vi "EXECUTION_UI_INIT.vi"(5 "Show Panel Label":bool, 7 "Layout":T1, 8 "error in (no error)":errorcluster, 10 "Execution Panels":refnum<vi>[](array[refnum]), 11 "Container Panel":refnum<vi>) -> (0 "error out":errorcluster, 2 "Execution Panels In Use":refnum<vi>[](array[refnum]))   [LabVIEW 2015, in "Execution.lvclass"]
uses:
  Execution.lvclass
  <vilib>/Utility/miscctls.llb/LVPointTypeDef.ctl
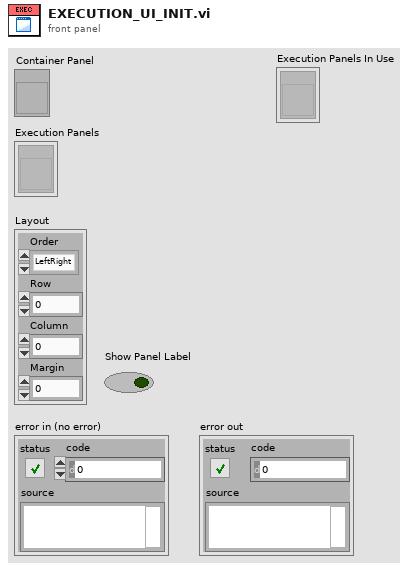
[diagram p1: front panel]
types:
  T1 = cluster{"Order":enum16{"LeftRight", "TopDown"}, "Row":i32, "Column":i32, "Margin":i32}
  T2 = enum16{"No Scaling", "Scale All Objects", "Scale Single Object"}
  T3 = typedef "LVPointTypeDef.ctl" = cluster{"Horizontal":i16, "Vertical":i16}
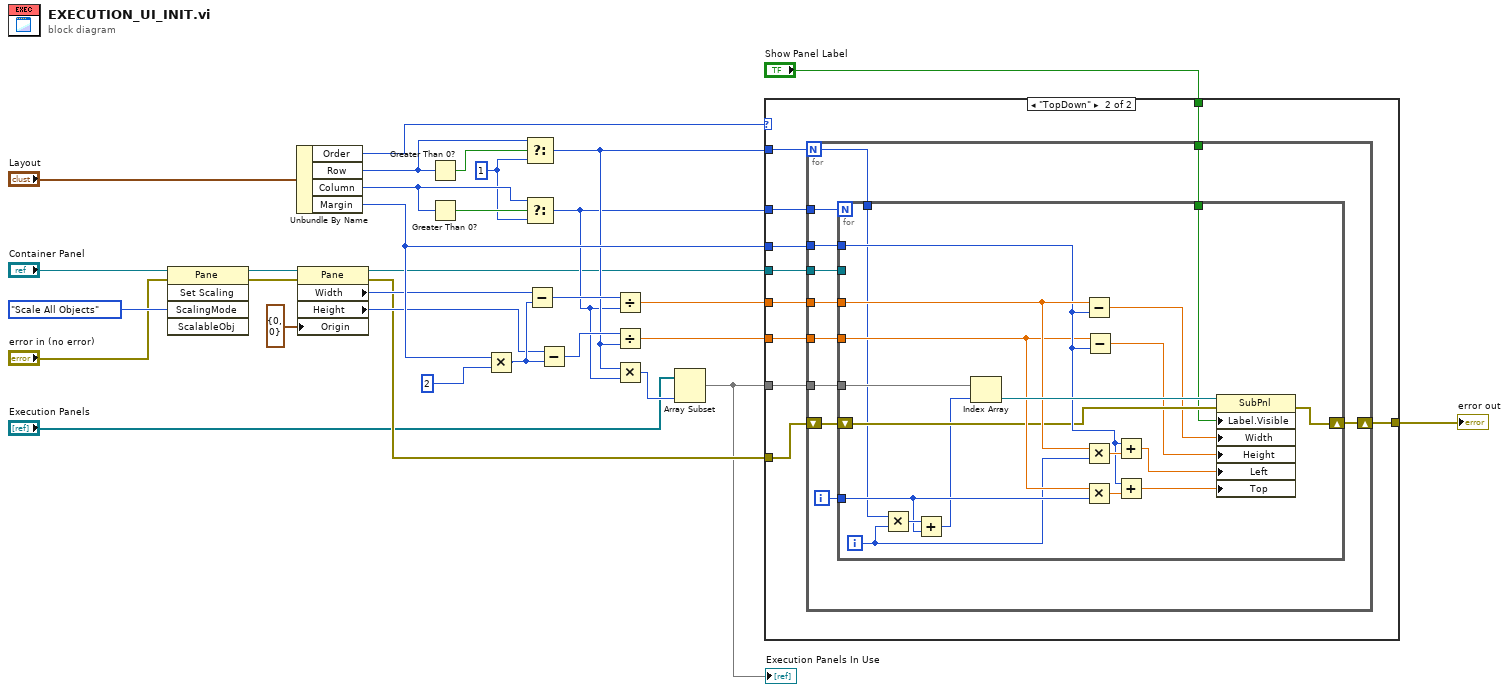
[diagram p0: block diagram]
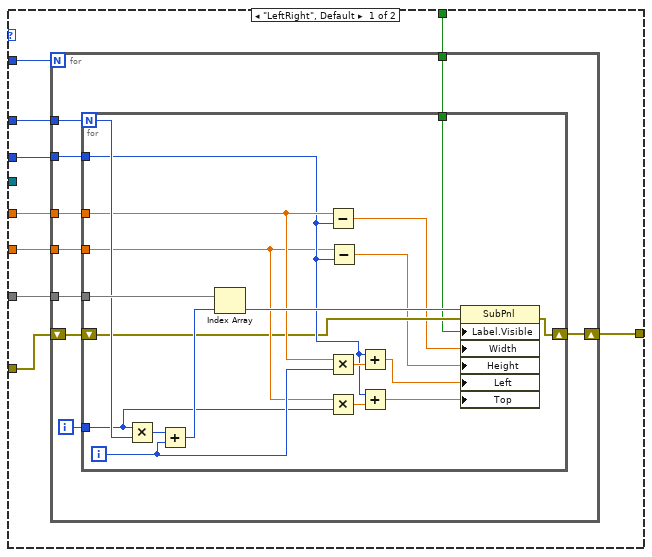
[diagram p2: hidden frame]
diagram:
  w13 = 1
  n1 = invoke class="Pane" method="Set Scaling"(reference="Container Panel", error in="error in (no error)", "ScalingMode"=T2."Scale All Objects" ("Scaling Mode")) -> (reference out=w2:refnum<vi>, error out=w3:errorcluster)  [unwired: 2 in, 3 out]
  n2 = Unbundle By Name("Layout") -> ("Order"=w30:enum16{"LeftRight", "TopDown"}, "Row"=w16:i32, "Column"=w14:i32, "Margin"=w31:i32)
  n3 = property class="Pane"(reference=w2, error in=w3, "Origin"=T3 {"Horizontal"=0, "Vertical"=0}) -> (reference out=w7:refnum<vi>, error out=w18:errorcluster, "Width"=w25:u32, "Height"=w26:u32)
  n4 = Greater Than 0?(x=w16) -> (x > 0?=w17:bool)
  n5 = Greater Than 0?(x=w14) -> (x > 0?=w15:bool)
  n6 = Multiply(x=w31, y=2) -> (x*y=w27:i32)
  n7 = Select(t=w16, s=w17, f=w13) -> (s? t:f=w12:i32)
  n8 = Select(t=w14, s=w15, f=w13) -> (s? t:f=w11:i32)
  n9 = Subtract(x=w25, y=w27) -> (x-y=w23:u32)
  n10 = Subtract(x=w26, y=w27) -> (x-y=w22:u32)
  n11 = Divide(x=w23, y=w11) -> (x/y=w19:dbl)
  n12 = Divide(x=w22, y=w12) -> (x/y=w20:dbl)
  n13 = Multiply(x=w12, y=w11) -> (x*y=w9:i32)
  n14 = Array Subset(array="Execution Panels", length=w9) -> (w10:refnum<vi>[])  [unwired: 1 in]
  "Execution Panels In Use" <- w10
  n15 = case shown="\"TopDown\"" w30 {
    tunnel: w19 -> [w40 w78]
    tunnel: w20 -> [w39 w77]
    tunnel: [w38 w76] -> w21
    tunnel: w10 -> [w37 w75]
    tunnel: w12 -> [w36 w74]
    tunnel: w11 -> [w35 w73]
    tunnel: w31 -> [w34 w72]
    tunnel: w18 -> [w33 w71]
    tunnel: "Show Panel Label" -> [w32 w70]
    tunnel: w7 -> [_ w69]
    frame "LeftRight", Default {
      n16 = for {
        N: w36 -> [_]
        tunnel: w37 -> [w49]
        tunnel: w40 -> [w48]
        tunnel: w39 -> [w47]
        tunnel: w35 -> [w45]
        tunnel: w34 -> [w43]
        shift-right: [w46] -> w38
        shift-left: w33 -> [w42]
        tunnel: w32 -> [w41]
        i -> [w44]
        n17 = for {
          N: w45 -> [w67]
          tunnel: w49 -> [w68]
          tunnel: w48 -> [w61]
          tunnel: w47 -> [w56]
          tunnel: w44 -> [w58]
          tunnel: w43 -> [w57]
          shift-right: [w63] -> w46
          shift-left: w42 -> [w55]
          tunnel: w41 -> [w50]
          i -> [w62]
          n18 = Multiply(x=w58, y=w67) -> (x*y=w66:i32)
          n19 = Add(x=w66, y=w62) -> (x+y=w65:i32)
          n20 = Index Array(array=w68, index=w65) -> (element=w64:refnum<vi>)
          n21 = Subtract(x=w61, y=w57) -> (x-y=w51:dbl)
          n22 = Multiply(x=w61, y=w62) -> (x*y=w60:dbl)
          n23 = Multiply(x=w56, y=w58) -> (x*y=w59:dbl)
          n24 = Subtract(x=w56, y=w57) -> (x-y=w52:dbl)
          n25 = Add(x=w57, y=w60) -> (x+y=w53:dbl)
          n26 = Add(x=w57, y=w59) -> (x+y=w54:dbl)
          n27 = property class="SubPnl"(reference=w64, error in=w55, "Label.Visible"=w50, "Width"=w51, "Height"=w52, "Left"=w53, "Top"=w54) -> (error out=w63:errorcluster)  [unwired: 1 out]
        }
      }
    }
    frame "TopDown" {
      n28 = for {
        N: w74 -> [w80]
        tunnel: w75 -> [w89]
        tunnel: w78 -> [w88]
        tunnel: w77 -> [w87]
        tunnel: w73 -> [w85]
        tunnel: w72 -> [w83]
        shift-right: [w86] -> w76
        shift-left: w71 -> [w82]
        tunnel: w70 -> [w81]
        tunnel: w69 -> [w79]
        i -> [w84]
        n29 = for {
          N: w85 -> [_]
          tunnel: w89 -> [w108]
          tunnel: w88 -> [w105]
          tunnel: w87 -> [w101]
          tunnel: w84 -> [w94]
          tunnel: w83 -> [w102]
          shift-right: [w90] -> w86
          shift-left: w82 -> [w100]
          tunnel: w81 -> [w95]
          tunnel: w80 -> [w91]
          tunnel: w79 -> [_]
          i -> [w93]
          n30 = Multiply(x=w91, y=w93) -> (x*y=w107:i32)
          n31 = Add(x=w107, y=w94) -> (x+y=w92:i32)
          n32 = Index Array(array=w108, index=w92) -> (element=w106:refnum<vi>)
          n33 = Subtract(x=w105, y=w102) -> (x-y=w96:dbl)
          n34 = Multiply(x=w105, y=w93) -> (x*y=w104:dbl)
          n35 = Multiply(x=w101, y=w94) -> (x*y=w103:dbl)
          n36 = Subtract(x=w101, y=w102) -> (x-y=w97:dbl)
          n37 = Add(x=w102, y=w104) -> (x+y=w98:dbl)
          n38 = Add(x=w102, y=w103) -> (x+y=w99:dbl)
          n39 = property class="SubPnl"(reference=w106, error in=w100, "Label.Visible"=w95, "Width"=w96, "Height"=w97, "Left"=w98, "Top"=w99) -> (error out=w90:errorcluster)  [unwired: 1 out]
        }
      }
    }
  }
  "error out" <- w21
